vi "Actor Core.vi"(8 "error in":errorcluster, 11 "SpectroscopyUI in":refnum<class "SpectroscopyUI.lvclass">) -> (0 "error out":errorcluster, 3 "Actor out":refnum<class "Actor.lvclass">)   [LabVIEW 2023, in "SpectroscopyUI.lvlib" / "SpectroscopyUI.lvclass"]
doc: "(<B>Filename</B>: Actor Framework.lvlib:Actor.lvclass:Actor Core.vi)\n\nReceives messages to the actor, reacts to them, and initiates any error handling that may shut the actor down.\n\nDescendant classes may override this VI to append parallel tasks for the actor to complete while it handles messages. Overrides use the Call Parent Class Method node."
uses:
  SpectroscopyUI.lvclass
  Applications/National Instruments/LabVIEW 2023 64-bit/vi.lib/ActorFramework/Actor/Actor.lvclass
  <vilib>/ActorFramework/Actor/Actor.lvclass
  SpectrSlitControl.ctl
  SpectroMirrorCtrl.ctl
  ConcreteClasses/ConcreteInstrumentClasses/SpectrometerClasses/Spectrometer_HRS_LV/HRS_Spectrometer/HRS_Spectrometer/HRS_Spectrometer.lvclass
  <vilib>/ActorFramework/Actor/Actor.lvclass/Actor.ctl
  <vilib>/ActorFramework/Message Enqueuer/Message Enqueuer.lvclass/Message Enqueuer.ctl
  SpectroscopyUI.lvclass/SpectroscopyUI.ctl
  ConcreteClasses/ConcreteInstrumentClasses/SpectrometerClasses/Spectrometer_HRS_LV/HRS_Spectrometer/HRS_Spectrometer Messages/Init Msg/Init Msg.lvclass/Init Msg.ctl
  ConcreteClasses/ConcreteInstrumentClasses/SpectrometerClasses/Spectrometer_HRS_LV/HRS_Spectrometer/HRS_Spectrometer Messages/GoToWavelength Msg/GoToWavelength Msg.lvclass/GoToWavelength Msg.ctl
  Interfaces/AbstractInstrumentClasses/Spectrometers_LV/Spectrometer Messages/SetMirror Msg/SetMirror Msg.lvclass/SetMirror Msg.ctl
  ConcreteClasses/ConcreteInstrumentClasses/SpectrometerClasses/Spectrometer_HRS_LV/HRS_Spectrometer/HRS_Spectrometer Messages/SetSlitwidth Msg/SetSlitwidth Msg.lvclass/SetSlitwidth Msg.ctl
  ConcreteClasses/ConcreteInstrumentClasses/SpectrometerClasses/Spectrometer_HRS_LV/HRS_Spectrometer/HRS_Spectrometer Messages/ChangeGrating Msg/ChangeGrating Msg.lvclass/ChangeGrating Msg.ctl
  <vilib>/ActorFramework/Message Enqueuer/Init from Existing Queue.vi
  <vilib>/ActorFramework/Message Enqueuer/Enqueue.vi
  ConcreteClasses/ConcreteInstrumentClasses/SpectrometerClasses/Spectrometer_HRS_LV/HRS_Spectrometer/HRS_Spectrometer Messages/DeInit Msg/DeInit Msg.lvclass
  Applications/National Instruments/LabVIEW 2023 64-bit/vi.lib/ActorFramework/Message/Message.lvclass
  ConcreteClasses/ConcreteInstrumentClasses/SpectrometerClasses/Spectrometer_HRS_LV/HRS_Spectrometer/HRS_Spectrometer Messages/Init Msg/Init Msg.lvclass
  ConcreteClasses/ConcreteInstrumentClasses/SpectrometerClasses/Spectrometer_HRS_LV/HRS_Spectrometer/HRS_Spectrometer Messages/QueryParameters Msg/QueryParameters Msg.lvclass
  ConcreteClasses/ConcreteInstrumentClasses/SpectrometerClasses/Spectrometer_HRS_LV/HRS_Spectrometer/HRS_Spectrometer Messages/GoToWavelength Msg/GoToWavelength Msg.lvclass
  Interfaces/AbstractInstrumentClasses/Spectrometers_LV/Spectrometer Messages/SetMirror Msg/SetMirror Msg.lvclass
  <vilib>/ActorFramework/Stop Msg/Stop Msg.lvclass
  ConcreteClasses/ConcreteInstrumentClasses/SpectrometerClasses/Spectrometer_HRS_LV/HRS_Spectrometer/HRS_Spectrometer Messages/SetSlitwidth Msg/SetSlitwidth Msg.lvclass
  ConcreteClasses/ConcreteInstrumentClasses/SpectrometerClasses/Spectrometer_HRS_LV/HRS_Spectrometer/HRS_Spectrometer Messages/ChangeGrating Msg/ChangeGrating Msg.lvclass
  <vilib>/ActorFramework/Message Priority Queue/Priority Enqueue.vi
  <vilib>/ActorFramework/Message Enqueuer/Message Enqueuer.lvclass
  SpectroscopyUI.lvlib
panel:
  out "Grating Out":u8
  in  "Set Grating":bool
  in  "Grating In":u8=1 min=1 max=3
  out "Front/Side Out":enum16{"FRONT", "SIDE"}(ring)
  out "Wavelength Out":dbl
  in  "Set Wavelength":bool
  in  "Wavelength In":dbl
  in  "Front/Side In":bool
  in  "Mirror":T1
  in  "Set Mirror Pos":bool
  in  "Slit":T2
  in  "Set Slitwidth":bool
  in  "Slitwidth In":dbl
  out "Slitwidth Out":u16
  in  "Connect":bool
  in  "VISA resource name":refnum<visa-resource-name>
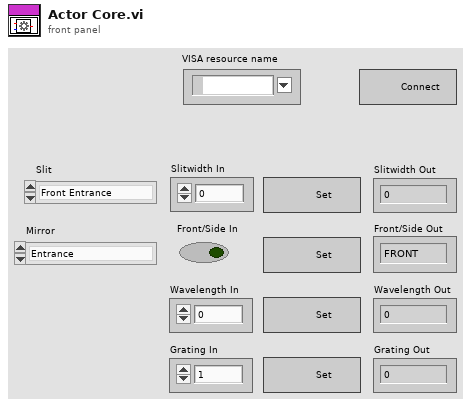
[diagram p1: front panel]
types:
  T1 = typedef "SpectroscopyUI.lvlib/SpectroMirrorCtrl.ctl" = enum16{"Entrance", "Exit"}
  T2 = typedef "SpectroscopyUI.lvlib/SpectrSlitControl.ctl" = enum16{"Front Entrance", "Side Entrance", "Front Exit", "Side Exit"}
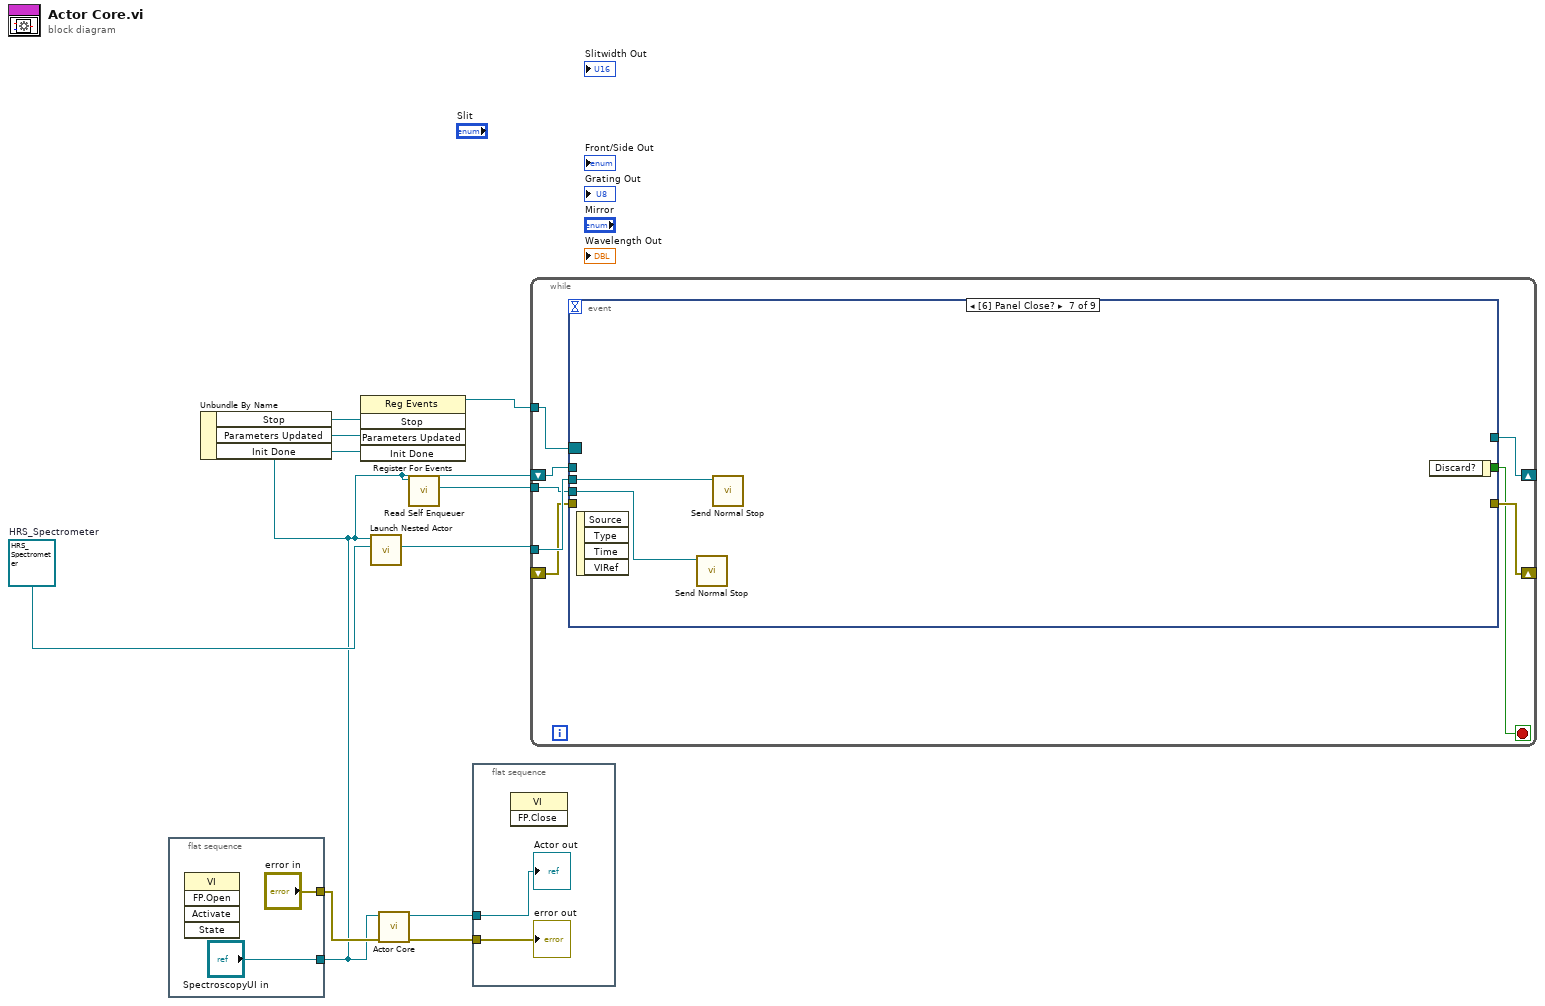
[diagram p0: block diagram]
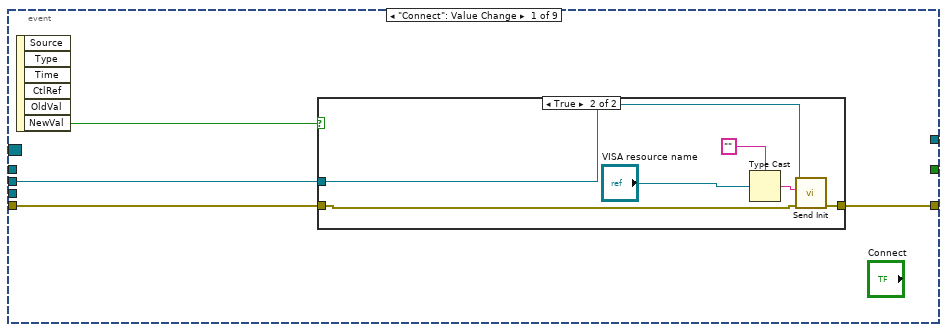
[diagram p2: hidden frame]
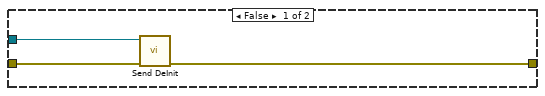
[diagram p3: hidden frame]
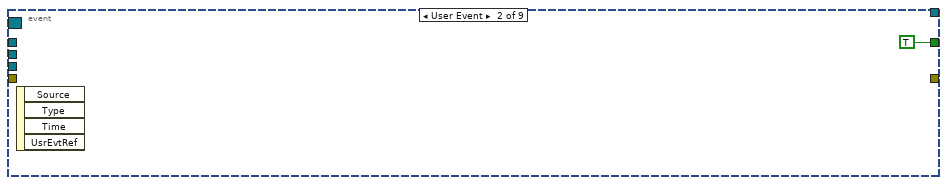
[diagram p4: hidden frame]
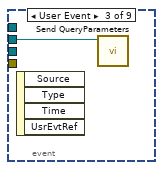
[diagram p5: hidden frame]
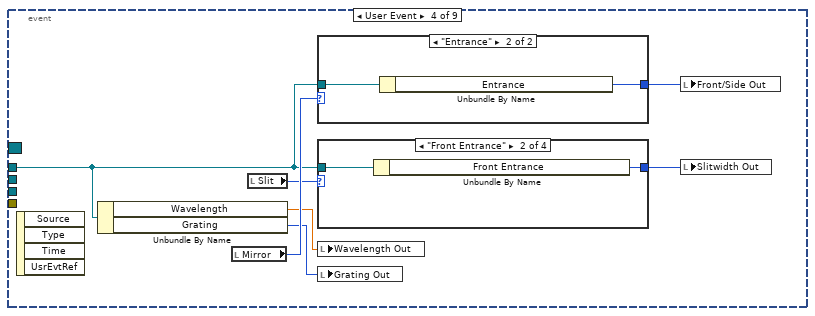
[diagram p6: hidden frame]
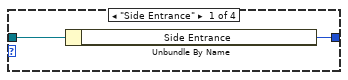
[diagram p7: hidden frame]
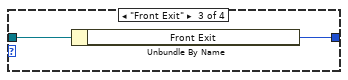
[diagram p8: hidden frame]
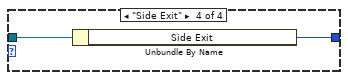
[diagram p9: hidden frame]
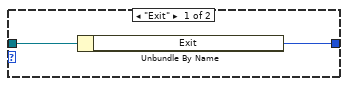
[diagram p10: hidden frame]
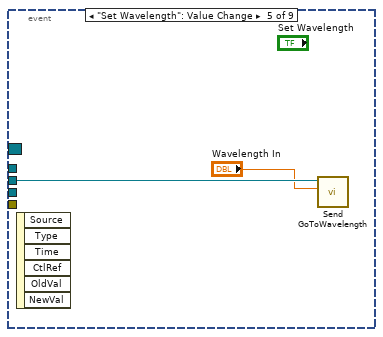
[diagram p11: hidden frame]
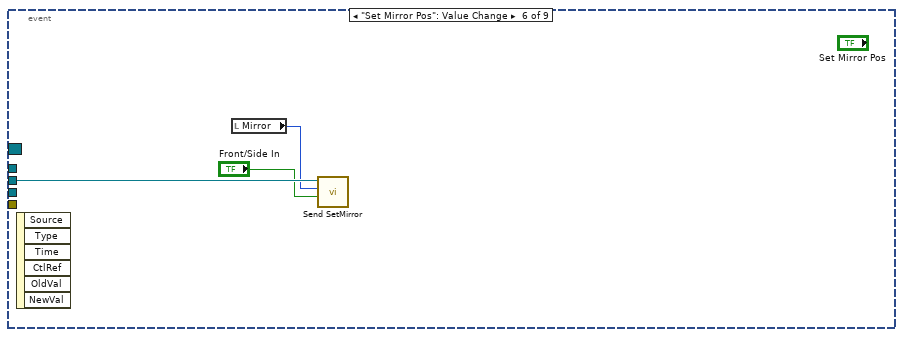
[diagram p12: hidden frame]
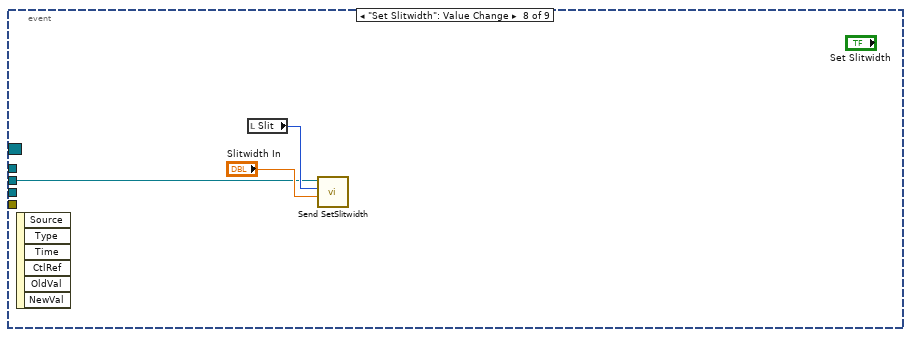
[diagram p13: hidden frame]
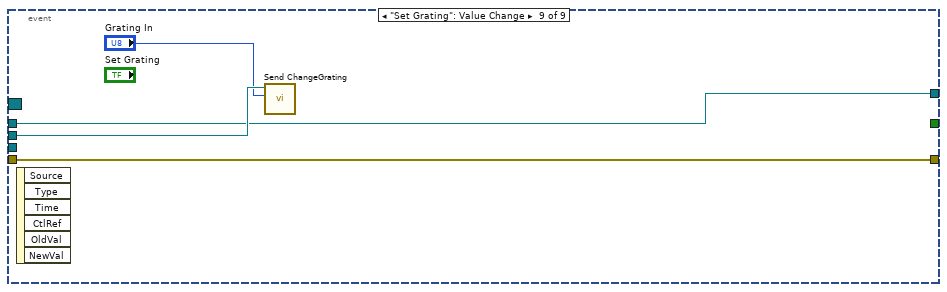
[diagram p14: hidden frame]
diagram:
  w7 = refnum<class "HRS_Spectrometer.lvclass"> refnum  # HRS_Spectrometer
  n1 = flat-sequence {
    tunnel: ["error in"] -> w9
    tunnel: ["SpectroscopyUI in"] -> w2
    frame #0 {
      n2 = invoke class="VI" method="FP.Open"() -> ()  [unwired: 5 in, 5 out]
    }
  }
  n3 = Unbundle By Name(w2) -> ("Stop"=w5:refnum<user-event>, "Parameters Updated"=w4:refnum<user-event>, "Init Done"=w3:refnum<user-event>)
  n4 = register-events(w5, w4, w3) -> (reference out=w6:refnum<event-registration>)  [unwired: 2 in, 1 out]
  n5 = call <vilib>:"Launch Nested Actor.vi"("Nested Actor"=w7, "Caller Actor in"=w2) -> ("Nested Actor's Enqueuer"=w8:refnum<class "Message Enqueuer.lvclass">)  [unwired: 7 in, 2 out]
  n6 = call-parent "Actor Core.vi"("error in"=w9, "Actor in"=w2) -> ("error out"=w11:errorcluster, "Actor out"=w10:refnum<class "Actor.lvclass">)  [unwired: 8 in]
  n7 = call <vilib>:"Read Self Enqueuer.vi"("Actor"=w2) -> ("Self Enqueuer"=w1:refnum<class "Message Enqueuer.lvclass">)  [unwired: 10 in]
  n8 = flat-sequence {
    tunnel: w11 -> [w15]
    tunnel: w10 -> [w14]
    frame #0 {
      n9 = invoke class="VI" method="FP.Close"() -> ()  [unwired: 3 in, 3 out]
      "error out" <- w15
      "Actor out" <- w14
    }
  }
  n10 = while {
    tunnel: w8 -> [w23]
    shift-right: [w21] -> _
    shift-left: _ -> [w22]
    tunnel: w6 -> [w20]
    shift-right: [w17] -> _
    shift-left: w2 -> [w18]
    tunnel: w1 -> [w16]
    stop <- w19 stop-if-true
    n11 = event shown="[6] Panel Close?" {
      selector: w20 -> [_ _ _ _ _ _ _ _ _]
      dyn-events: _ -> [_ _ _ _ _ _ _ _ _]
      timeout: _ -> [_ _ _ _ _ _ _ _ _]
      tunnel: w23 -> [w27 _ w38 _ w59 w62 w64 w65 w71]
      tunnel: w22 -> [w26 _ _ _ _ _ _ _ w69]
      tunnel: [w25 _ _ _ _ _ _ _ w69] -> w21
      tunnel: [_ TRUE _ _ _ _ _ _ _] -> w19
      tunnel: w18 -> [_ _ _ w41 _ _ _ _ w68]
      tunnel: [_ _ _ _ _ _ _ _ w68] -> w17
      tunnel: w16 -> [_ _ _ _ _ _ w63 _ _]
      event "Connect": Value Change {
        n12 = event-data() -> ("NewVal"=w24:bool)  [unwired: 1 in, 5 out]
        n13 = case shown="True" w24 {
          tunnel: w27 -> [w30 w36]
          tunnel: w26 -> [w29 w32]
          tunnel: [w28 w31] -> w25
          frame False {
            n14 = call "Send DeInit.vi"("error in (no error)"=w29, "Message Enqueuer"=w30) -> ("error out"=w28:errorcluster)  [unwired: 8 in, 1 out]
          }
          frame True {
            n15 = Type Cast(type="" ("Address"), x="VISA resource name") -> (*(type *) &x=w33:string)
            n16 = call "Send Init.vi"("error in (no error)"=w32, "Address"=w33, "Message Enqueuer"=w36) -> ("error out"=w31:errorcluster)  [unwired: 7 in, 1 out]
          }
        }
      }
      event User Event {
        n17 = event-data() -> ()  [unwired: 1 in, 4 out]
      }
      event User Event {
        n18 = event-data() -> ()  [unwired: 1 in, 4 out]
        n19 = call "Send QueryParameters.vi"("Message Enqueuer"=w38) -> ()  [unwired: 9 in, 2 out]
      }
      event User Event {
        n20 = event-data() -> ()  [unwired: 1 in, 4 out]
        n21 = Unbundle By Name(w41) -> ("Wavelength"=w40:dbl, "Grating"=w39:enum16{"Mirror", "1200 g/mm", "1800 g/mm"})
        n22 = local read "Mirror"() -> (w45:T1)
        n23 = local read "Slit"() -> (w43:T2)
        n24 = case shown="\"Entrance\"" w45 {
          tunnel: w41 -> [w55 w57]
          tunnel: [w54 w56] -> w44
          frame "Exit" {
            n25 = Unbundle By Name(w55) -> ("Exit"=w54:enum16{"FRONT", "SIDE"})
          }
          frame "Entrance" {
            n26 = Unbundle By Name(w57) -> ("Entrance"=w56:enum16{"FRONT", "SIDE"})
          }
        }
        n27 = case shown="\"Front Entrance\"" w43 {
          tunnel: [w47 w49 w51 w53] -> w42
          tunnel: w41 -> [w46 w48 w50 w52]
          frame "Side Entrance" {
            n28 = Unbundle By Name(w46) -> ("Side Entrance"=w47:u16)
          }
          frame "Front Entrance" {
            n29 = Unbundle By Name(w48) -> ("Front Entrance"=w49:u16)
          }
          frame "Front Exit" {
            n30 = Unbundle By Name(w50) -> ("Front Exit"=w51:u16)
          }
          frame "Side Exit" {
            n31 = Unbundle By Name(w52) -> ("Side Exit"=w53:u16)
          }
        }
        n32 = local write "Wavelength Out"(w40) -> ()
        n33 = local write "Grating Out"(w39) -> ()
        n34 = local write "Front/Side Out"(w44) -> ()
        n35 = local write "Slitwidth Out"(w42) -> ()
      }
      event "Set Wavelength": Value Change {
        n36 = event-data() -> ()  [unwired: 1 in, 6 out]
        n37 = call "Send GoToWavelength.vi"("Wavelength"="Wavelength In", "Message Enqueuer"=w59) -> ()  [unwired: 8 in, 2 out]
      }
      event "Set Mirror Pos": Value Change {
        n38 = event-data() -> ()  [unwired: 1 in, 6 out]
        n39 = local read "Mirror"() -> (w60:T1)
        n40 = call "Send SetMirror.vi"("Front/Side"="Front/Side In", "Mirror"=w60, "Message Enqueuer"=w62) -> ()  [unwired: 7 in, 2 out]
      }
      event Panel Close? {
        n41 = event-data() -> ()  [unwired: 1 in, 4 out]
        n42 = call <vilib>:"Send Normal Stop.vi"("Message Enqueuer"=w63) -> ()  [unwired: 10 in, 1 out]
        n43 = call <vilib>:"Send Normal Stop.vi"("Message Enqueuer"=w64) -> ()  [unwired: 10 in, 1 out]
        n44 = event-data() -> ()  [unwired: 2 in, 1 out]
      }
      event "Set Slitwidth": Value Change {
        n45 = event-data() -> ()  [unwired: 1 in, 6 out]
        n46 = local read "Slit"() -> (w66:T2)
        n47 = call "Send SetSlitwidth.vi"("Slitwidth"="Slitwidth In", "Slit"=w66, "Message Enqueuer"=w65) -> ()  [unwired: 7 in, 2 out]
      }
      event "Set Grating": Value Change {
        n48 = event-data() -> ()  [unwired: 1 in, 6 out]
        n49 = call "Send ChangeGrating.vi"("Grating"="Grating In", "Message Enqueuer"=w71) -> ()  [unwired: 8 in, 2 out]
      }
    }
  }
